vi "Create Enumerator(冲突时的文件备份2013-03-27 14-07-47).vi"(8 "error in (no error)":errorcluster caption="错误输入（无错误）", 10 "path":string, 11 "ManagementClass 输入":refnum<class "ManagementClass.lvclass"> caption="DNL_LabVIEW Object in") -> (0 "error out":errorcluster caption="错误输出", 3 "ManagementClass 输出":refnum<class "ManagementClass.lvclass"> caption="DNL_LabVIEW Object out")   [LabVIEW 2012, in "ManagementClass.lvclass"]
uses:
  ManagementClass.lvclass
  ManagementClass.lvclass/ManagementClass.ctl
  System.Management
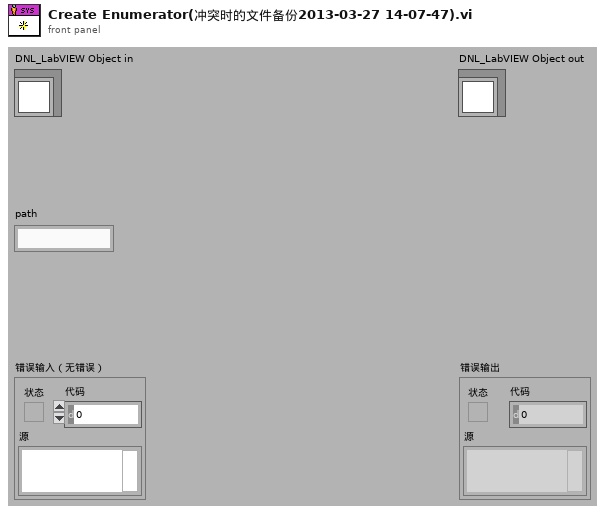
[diagram p1: front panel]
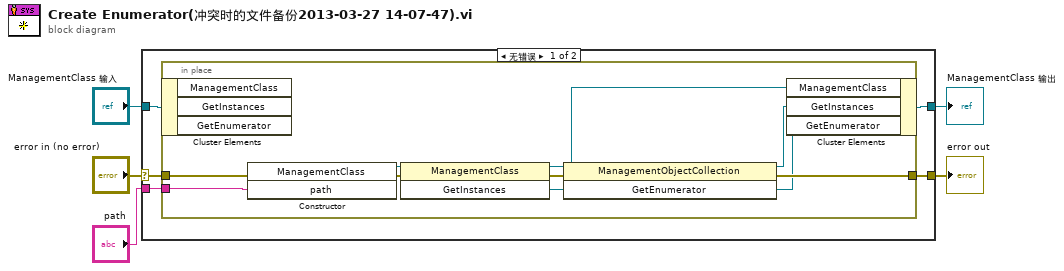
[diagram p0: block diagram]
diagram:
  n1 = case shown="无错误" "error in (no error)" {
    selector: "error in (no error)" -> [w8 w22]
    tunnel: [w7 w22] -> w4
    tunnel: [w6 w21] -> w2
    tunnel: "ManagementClass 输入" -> [w10 w21]
    tunnel: "path" -> [w9 _]
    frame No Error {
      n2 = in-place {
        in-place-border: w9 -> [w17]
        in-place-border: w8 -> [w16]
        in-place-border: [w14] -> w7
        n3 = in-place-cluster #1(w10) -> ()  [unwired: 3 out]
        n4 = constructor class="ManagementClass"(error in=w16, "path"=w17) -> (reference out=w18:refnum<k24>, error out=w19:errorcluster)  [unwired: 2 in, 2 out]
        n5 = invoke class="ManagementClass" method="GetInstances"(reference=w18, error in=w19) -> (reference out=w13:refnum<k24>, error out=w15:errorcluster, "GetInstances"=w20:refnum<k24>)  [unwired: 1 in]
        n6 = invoke class="ManagementObjectCollection" method="GetEnumerator"(reference=w20, error in=w15) -> (reference out=w12:refnum<k24>, error out=w14:errorcluster, "GetEnumerator"=w11:refnum<k24>)  [unwired: 1 in]
        n7 = in-place-cluster #1("ManagementClass"=w13, "GetInstances"=w12, "GetEnumerator"=w11) -> (w6:refnum<class "ManagementClass.lvclass">)
      }
    }
    frame Error {
    }
  }
  "error out" <- w4
  "ManagementClass 输出" <- w2
